vi "String EW.vi"(11 "Data In":string) -> (3 "Data Out":string)   [LabVIEW 2016]
uses:
  Core/Assert API Components/Failure Actions.ctl
  Core/Assert API Components/Assert API Components.lvlib
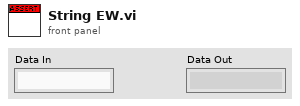
[diagram p1: front panel]
types:
  T1 = typedef "Assert API Components.lvlib/Failure Actions.ctl" = enum16{"None", "Log To File", "Pause Execution", "Abort Execution"}
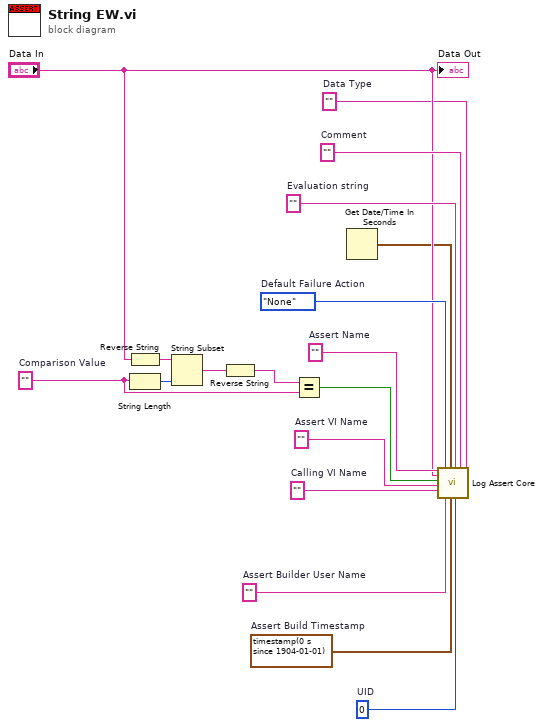
[diagram p0: block diagram]
diagram:
  w1 = 0  # UID
  w3 = ""  # Assert VI Name
  w4 = ""  # Calling VI Name
  w5 = ""  # Data Type
  w6 = ""  # Assert Builder User Name
  w7 = timestamp(0 s since 1904-01-01)  # Assert Build Timestamp
  w16 = ""  # Comment
  w15 = ""  # Evaluation string
  w17 = Failure_Actions."None"  # Default Failure Action
  w18 = ""  # Assert Name
  w11 = ""  # Comparison Value
  n1 = Reverse String(1:"Data In") -> (0:w9:string)
  n2 = String Length(string=w11) -> (length=w13:i32)
  n3 = String Subset(string=w9, length (rest)=w13) -> (substring=w12:string)  [unwired: 1 in]
  n4 = Reverse String(1:w12) -> (0:w8:string)
  n5 = Equal?(x=w8, y=w11) -> (x = y?=w10:bool)
  n6 = Get Date/Time In Seconds() -> (seconds since 1Jan1904=w2:timestamp)
  n7 = call "Log Assert Core.vi"("Assert Name"=w18, "Data Value"="Data In", "Status"=w10, "Assert VI Name"=w3, "Calling VI Name"=w4, "Failure Action"=w17, "Assert Builder User Name"=w6, "Last Update"=w2, "Assert Build Timestamp"=w7, "Evaluation String"=w15, "Assert VI UID"=w1, "Comment"=w16, "Data Type"=w5) -> ()  [unwired: 7 in]
  "Data Out" <- "Data In"
